vi "startEditor.vi"(8 "error in (no error)":errorcluster, 9 "deviceDataBase":refnum<class "deviceDataBase.lvclass">, 10 "ScriptEdEvents":refnum<class "ScriptEdEvents.lvclass">, 11 "ScriptEditorV2 in":refnum<class "ScriptEditorV2.lvclass">) -> (0 "error out":errorcluster, 3 "ScriptEditorV2 out":refnum<class "ScriptEditorV2.lvclass">)   [LabVIEW 2009, in "Views.lvlib" / "ScriptEditor.lvlib" / "ScriptEditorV2.lvclass"]
uses:
  ScriptEditorV2.lvclass
  ScriptEdEvents/ScriptEdEvents.lvclass
  Tools/DatabaseHelpers/DbConnection/DeviceDataBase/deviceDataBase.lvclass
  Tools/Scripting/ScriptingEvent/ScriptEventList/ScriptEventList.lvclass
  ScriptEditorV2.lvclass/ScriptEditorV2.ctl
  Tools/Filing/FileSystem/FileSystem.lvclass
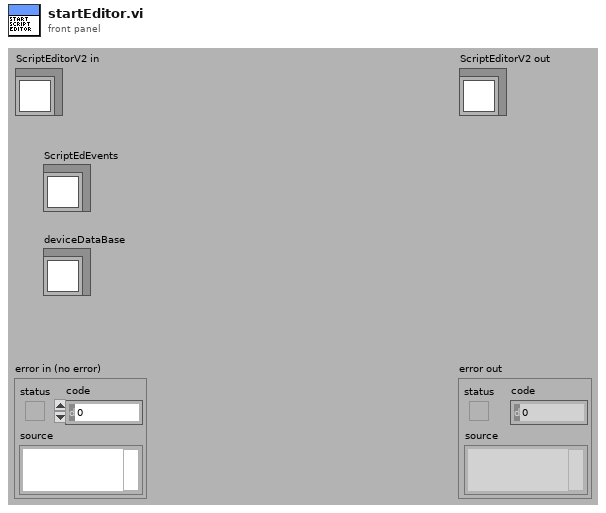
[diagram p1: front panel]
types:
  T1 = enum32{"Invalid", "Standard", "Closed", "Hidden", "Minimized", "Maximized"}
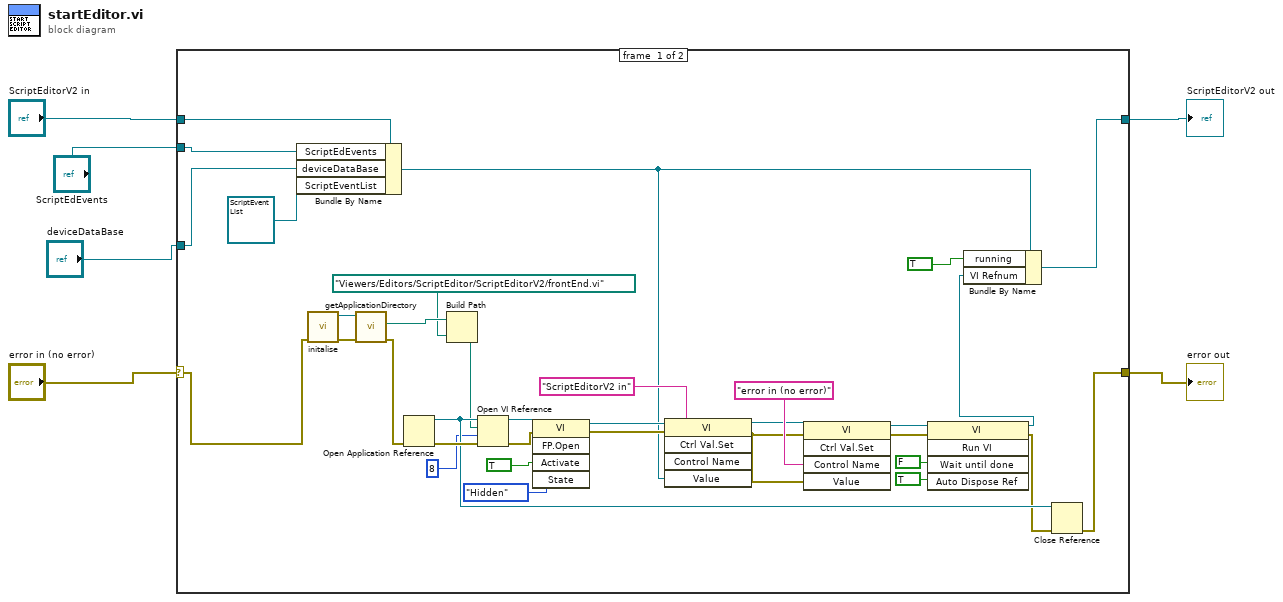
[diagram p0: block diagram]
diagram:
  n1 = case shown="No Error" "error in (no error)" {
    selector: "error in (no error)" -> [w13 w42]
    tunnel: [w32 w42] -> w5
    tunnel: "ScriptEditorV2 in" -> [w22 w41]
    tunnel: [w20 w41] -> w6
    tunnel: "deviceDataBase" -> [w23 _]
    tunnel: "ScriptEdEvents" -> [w9 _]
    frame #0 {
      n2 = Bundle By Name(cluster=w22, "ScriptEdEvents"=w9, "deviceDataBase"=w23, "ScriptEventList"=refnum<class "ScriptEventList.lvclass"> refnum) -> (w18:refnum<class "ScriptEditorV2.lvclass">)
      n3 = call "initalise.vi"("error in (no error)"=w13) -> ("error out"=w15:errorcluster, "FileSystem out"=w14:refnum<class "FileSystem.lvclass">)  [unwired: 9 in]
      n4 = call-dynamic "getApplicationDirectory.vi"("error in (no error)"=w15, "FileSystem.lvclass in"=w14) -> ("error out"=w12:errorcluster, "ApplicationDirectory"=w17:path)  [unwired: 7 in, 1 out]
      n5 = Open Application Reference(8:w12) -> (0:w37:errorcluster, 3:w34:refnum<vi>)  [unwired: 3 in]
      n6 = Build Path(base path=w17, name or relative path=path "Viewers/Editors/ScriptEditor/ScriptEditorV2/frontEnd.vi" ("vi path")) -> (appended path=w11:path)
      n7 = Open VI Reference(application reference (local)=w34, vi path=w11, options=8, error in (no error)=w37) -> (vi reference=w29:refnum<vi>, error out=w28:errorcluster)  [unwired: 2 in]
      n8 = invoke class="VI" method="FP.Open"(reference=w29, error in=w28, "Activate"=TRUE, "State"=T1."Hidden") -> (reference out=w27:refnum<vi>, error out=w26:errorcluster)  [unwired: 1 in, 3 out]
      n9 = invoke class="VI" method="Ctrl Val.Set"(reference=w27, error in=w26, "Control Name"="ScriptEditorV2 in", "Value"=w18) -> (reference out=w36:refnum<vi>, error out=w35:errorcluster)  [unwired: 1 in, 3 out]
      n10 = invoke class="VI" method="Ctrl Val.Set"(reference=w36, error in=w35, "Control Name"="error in (no error)", "Value"=w35) -> (reference out=w31:refnum<vi>, error out=w30:errorcluster)  [unwired: 1 in, 3 out]
      n11 = invoke class="VI" method="Run VI"(reference=w31, error in=w30, "Wait until done"=FALSE, "Auto Dispose Ref"=TRUE) -> (reference out=w7:refnum<vi>, error out=w33:errorcluster)  [unwired: 1 in, 3 out]
      n12 = Bundle By Name(cluster=w18, "running"=TRUE, "VI Refnum"=w7) -> (w20:refnum<class "ScriptEditorV2.lvclass">)
      n13 = Close Reference(reference=w34, error in (no error)=w33) -> (error out=w32:errorcluster)
    }
    frame #1 {
    }
  }
  "error out" <- w5
  "ScriptEditorV2 out" <- w6
